vi "Globals.vi"() -> ()   [LabVIEW 2017]
panel:
  in  "nosnobchanged":bool
  in  "cam_sel":u8
  in  "nob":u32
  in  "dioden 2":u16[][](array[numeric])
  in  "dioden 1":u16[][](array[numeric])
  in  "exp time":dbl
  in  "nos":u32
  in  "PIXEL":u32
  in  "boards":u32
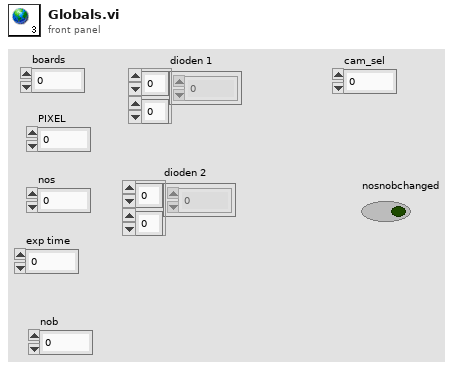
[diagram p1: front panel]
diagram:
